vi "Map To Driver.vi"(0 "ResourceEnumerator in":refnum<class "ResourceEnumerator.lvclass">, 5 "Driver Name":string, 11 "error in (no error)":errorcluster) -> (4 "ResourceEnumerator out":refnum<class "ResourceEnumerator.lvclass">, 6 "Driver":refnum<class "Driver.lvclass">, 15 "error out":errorcluster)   [LabVIEW 2023]
doc: "Passed an alias or canonical name it returns a concrete Driver (Instrument) instance or raises error 200 if no match found.\n\nMust be implemented by a subclass."
uses:
  ResourceEnumerator.lvclass/ResourceEnumerator.ctl
  ResourceEnumerator.lvclass
  DMM6500/DMM6500.lvclass
  HMC8043/HMC8043.lvclass
  SDS1104X-E/SDS1104X-E.lvclass
  SDG1032X/SDG1032X.lvclass
  \\Mac\Home/Documents/LabVIEW Data/ProjectTemplates/Source/HAF/Driver/Driver.lvclass
  \\Mac\Home/Documents/LabVIEW Data/ProjectTemplates/Source/HAF/DMM6500/DMM6500.lvclass
  \\Mac\Home/Documents/LabVIEW Data/ProjectTemplates/Source/HAF/HMC8043/HMC8043.lvclass
  \\Mac\Home/Documents/LabVIEW Data/ProjectTemplates/Source/HAF/SDS1104X-E/SDS1104X-E.lvclass
  \\Mac\Home/Documents/LabVIEW Data/ProjectTemplates/Source/HAF/SDG1032X/SDG1032X.lvclass
  Driver/Driver.lvclass
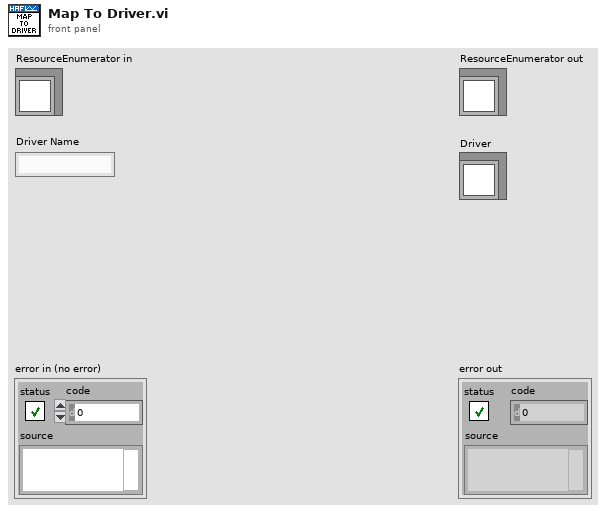
[diagram p1: front panel]
types:
  T1 = typedef "HAF.lvlib/Resource Structure.ctl" = cluster{"Alias":string, "Canonical Name":string}
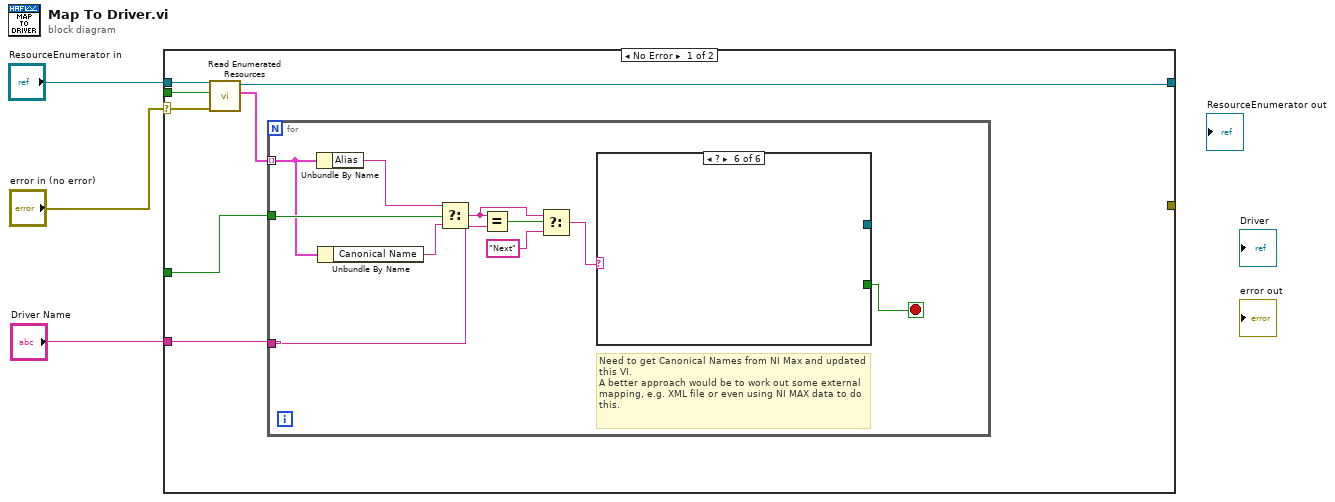
[diagram p0: block diagram]
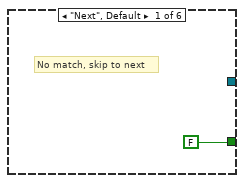
[diagram p2: hidden frame]
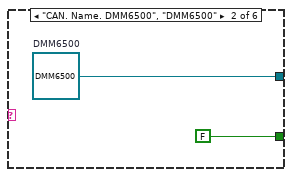
[diagram p3: hidden frame]
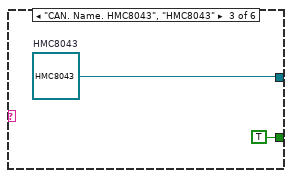
[diagram p4: hidden frame]
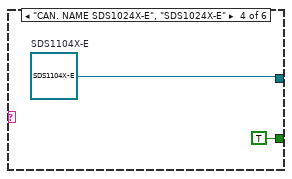
[diagram p5: hidden frame]
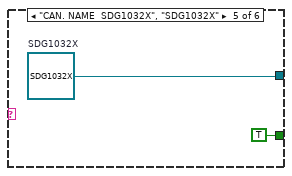
[diagram p6: hidden frame]
diagram:
  n1 = case shown="No Error" "error in (no error)" {
    selector: "error in (no error)" -> [w10 w32]
    tunnel: "ResourceEnumerator in" -> [w12 w33]
    tunnel: [w9 w33] -> _
    tunnel: [_ w32] -> _
    tunnel: [w11 _] -> w3
    tunnel: [w7 _] -> w2
    tunnel: "Driver Name" -> [w6 _]
    frame No Error {
      n2 = call-dynamic "Read Enumerated Resources.vi"("error in (no error)"=w10, "Refresh"=w11, "AbstractResourceEnumerator in"=w12) -> ("Enumerated Resources"=w8:T1[], "AbstractResourceEnumerator out"=w9:refnum<class "ResourceEnumerator.lvclass">)  [unwired: 6 in, 1 out]
      n3 = for {
        tunnel: w8 -> [w20] mode=indexing
        tunnel: w7 -> [w21]
        tunnel: w6 -> [w18]
        stop <- w13 stop-if-true
        # "Need to get Canonical Names from NI Max and updated this VI.\nA better approach would be to work out some external mapping, e.g. XML file or even using NI MAX data to do this."
        n4 = Unbundle By Name(w20) -> ("Alias"=w22:string)
        n5 = Unbundle By Name(w20) -> ("Canonical Name"=w19:string)
        n6 = Select(t=w22, s=w21, f=w19) -> (s? t:f=w16:string)
        n7 = Equal?(x=w16, y=w18) -> (x = y?=w17:bool)
        n8 = Select(t=w16, s=w17, f="Next") -> (s? t:f=w14:string)
        n9 = case w14 {
          tunnel: [_ w25 w27 w29 w31 _] -> _
          tunnel: [FALSE FALSE TRUE TRUE TRUE _] -> w13
          frame "Next", Default {
            # "No match, skip to next"
          }
          frame "CAN. Name. DMM6500", "DMM6500" {
            w25 = refnum<class "DMM6500.lvclass"> refnum  # DMM6500
          }
          frame "CAN. Name. HMC8043", "HMC8043" {
            w27 = refnum<class "HMC8043.lvclass"> refnum  # HMC8043
          }
          frame "CAN. NAME SDS1024X-E", "SDS1024X-E" {
            w29 = refnum<class "SDS1104X-E.lvclass"> refnum  # SDS1104X-E
          }
          frame "CAN. NAME  SDG1032X", "SDG1032X" {
            w31 = refnum<class "SDG1032X.lvclass"> refnum  # SDG1032X
          }
          frame ? {
          }
        }
      }
    }
    frame Error {
    }
  }
